vi "pc_find_single_peak.vi"(8 "error in (no error)":errorcluster, 11 "Plots in":refnum<class "Plots.lvclass">) -> (0 "error out":errorcluster, 3 "Plots out":refnum<class "Plots.lvclass">)   [LabVIEW 2017, in "Plots.lvclass"]
doc: "find single peak in plot data by finding the half heights of the flanks.\n\nPlot data and threshold are all saved in the PlotObjects private properties.\nFound peak centers, half heights are also saved in the private properties."
uses:
  Plots.lvclass
panel:
  out "peak found?":bool
  out "pc_right-half":dbl
  out "pc_center":dbl
  out "pc_left-half":dbl
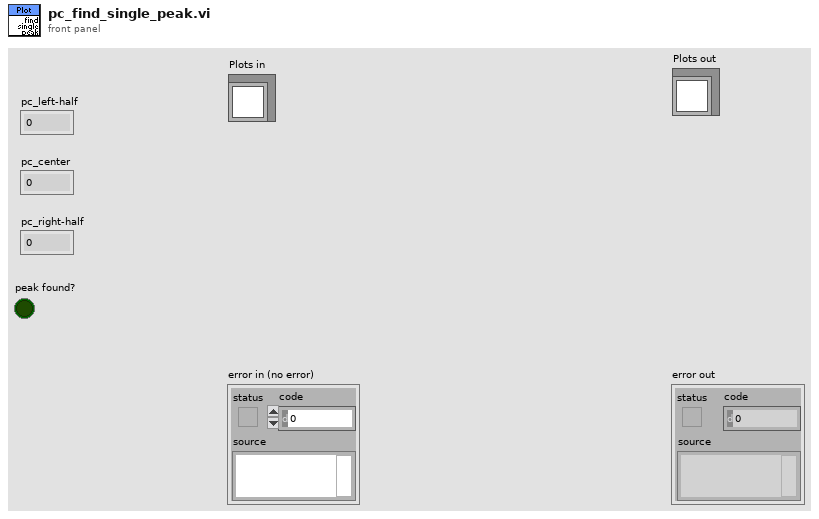
[diagram p1: front panel]
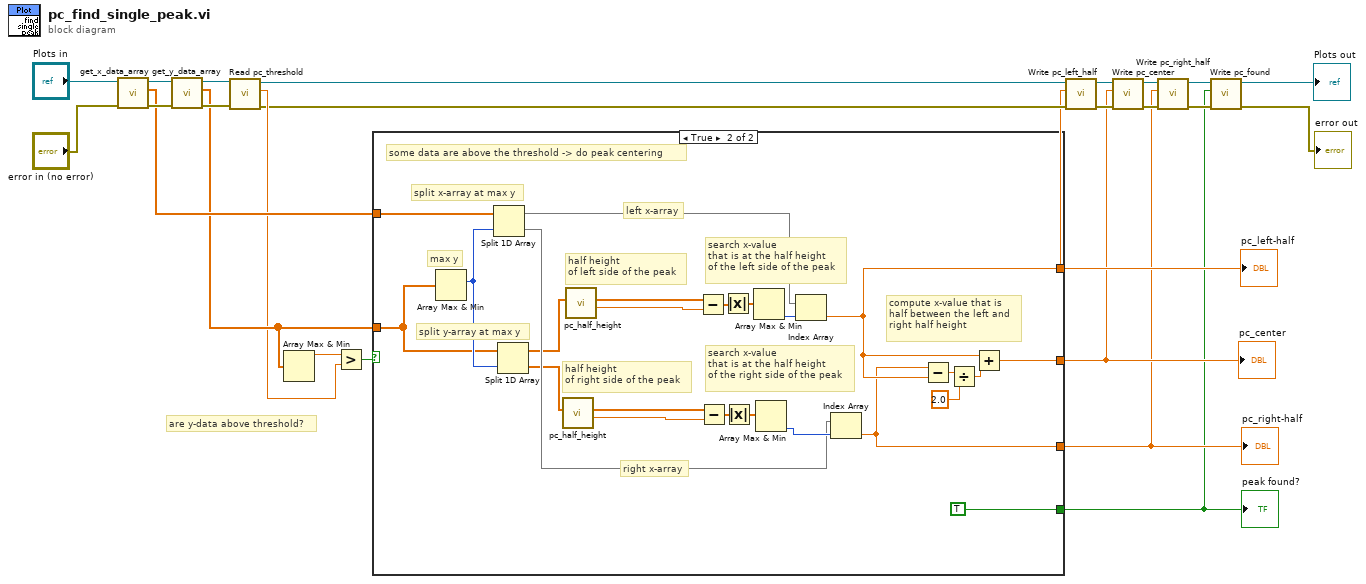
[diagram p0: block diagram]
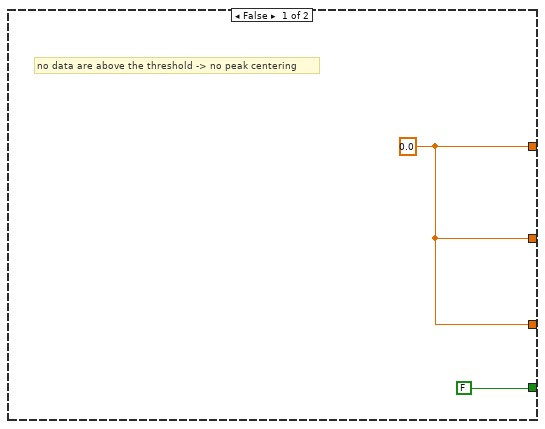
[diagram p2: hidden frame]
diagram:
  # "are y-data above threshold?"
  n1 = call-dynamic "get_x_data_array.vi"("error in (no error)"="error in (no error)", "Plots in"="Plots in") -> ("error out"=w20:errorcluster, "x-Array"=w17:dbl[], "Plots out"=w21:refnum<class "Plots.lvclass">)  [unwired: 7 in]
  n2 = call-dynamic "get_y_data_array.vi"("error in (no error)"=w20, "Plots in"=w21) -> ("error out"=w18:errorcluster, "y-Array"=w16:dbl[], "Plots out"=w19:refnum<class "Plots.lvclass">)  [unwired: 7 in]
  n3 = call-dynamic "Read pc_threshold.vi"("error in (no error)"=w18, "Plots in"=w19) -> ("error out"=w13:errorcluster, "pc_threshold"=w15:dbl, "Plots out"=w14:refnum<class "Plots.lvclass">)  [unwired: 7 in]
  n4 = Array Max & Min(array=w16) -> (max value=w24:dbl)  [unwired: 3 out]
  n5 = Greater?(x=w24, y=w15) -> (0:w25:bool)
  n6 = case shown="True" w25 {
    tunnel: w17 -> [_ w46]
    tunnel: [w27 w42] -> w8
    tunnel: [w27 w38] -> w7
    tunnel: [w27 w37] -> w6
    tunnel: w16 -> [_ w34]
    tunnel: [FALSE TRUE] -> w3
    frame False {
      w27 = 0.0
      # "no data are above the threshold -> no peak centering"
    }
    frame True {
      # "compute x-value that is\nhalf between the left and\nright half height"
      # "search x-value\nthat is at the half height\nof the right side of the peak"
      # "search x-value\nthat is at the half height\nof the left side of the peak"
      # "right x-array"
      # "left x-array"
      # "half height\nof right side of the peak"
      # "split y-array at max y"
      # "some data are above the threshold -> do peak centering"
      # "split x-array at max y"
      # "half height\nof left side of the peak"
      # "max y"
      n7 = Array Max & Min(array=w34) -> (max index (indices)=w45:i32)  [unwired: 3 out]
      n8 = Split 1D Array(array=w46, index=w45) -> (first subarray=w49:dbl[], second subarray=w50:dbl[])
      n9 = Split 1D Array(array=w34, index=w45) -> (first subarray=w36:dbl[], second subarray=w43:dbl[])
      n10 = call "pc_half_height.vi"("y-data in"=w43) -> ("half height out"=w44:dbl, "y-data out"=w48:dbl[])  [unwired: 8 in, 1 out]
      n11 = call "pc_half_height.vi"("y-data in"=w36) -> ("half height out"=w29:dbl, "y-data out"=w47:dbl[])  [unwired: 8 in, 1 out]
      n12 = Subtract(x=w47, y=w29) -> (x-y=w30:dbl[])
      n13 = Subtract(x=w48, y=w44) -> (x-y=w33:dbl[])
      n14 = Absolute Value(x=w30) -> (abs(x)=w31:dbl[])
      n15 = Absolute Value(x=w33) -> (abs(x)=w32:dbl[])
      n16 = Array Max & Min(array=w31) -> (min index (indices)=w35:i32)  [unwired: 3 out]
      n17 = Array Max & Min(array=w32) -> (min index (indices)=w51:i32)  [unwired: 3 out]
      n18 = Index Array(array=w49, index=w35) -> (element=w42:dbl)
      n19 = Index Array(array=w50, index=w51) -> (element=w37:dbl)
      n20 = Subtract(x=w37, y=w42) -> (x-y=w39:dbl)
      n21 = Divide(x=w39, y=2.0) -> (x/y=w41:dbl)
      n22 = Add(x=w42, y=w41) -> (x+y=w38:dbl)
    }
  }
  "pc_left-half" <- w8
  "pc_center" <- w7
  "pc_right-half" <- w6
  "peak found?" <- w3
  n23 = call-dynamic "Write pc_left_half.vi"("error in (no error)"=w13, "pc_left_half"=w8, "Plots in"=w14) -> ("error out"=w11:errorcluster, "Plots out"=w12:refnum<class "Plots.lvclass">)  [unwired: 7 in]
  n24 = call-dynamic "Write pc_center.vi"("error in (no error)"=w11, "pc_center"=w7, "Plots in"=w12) -> ("error out"=w9:errorcluster, "Plots out"=w10:refnum<class "Plots.lvclass">)  [unwired: 7 in]
  n25 = call-dynamic "Write pc_right_half.vi"("error in (no error)"=w9, "pc_right_half"=w6, "Plots in"=w10) -> ("error out"=w4:errorcluster, "Plots out"=w5:refnum<class "Plots.lvclass">)  [unwired: 7 in]
  n26 = call-dynamic "Write pc_found.vi"("error in (no error)"=w4, "pc_found"=w3, "Plots in"=w5) -> ("error out"=→"error out":errorcluster, "Plots out"=→"Plots out":refnum<class "Plots.lvclass">)  [unwired: 7 in]
